vi "标准波形子VI.vi"(4 "采样信息":cluster{"Fs":dbl, "#s":dbl}={"Fs"=1000.0, "#s"=1000.0} {"Fs" format="%.2p"}, 5 "幅值":dbl, 6 "formula":string="sin(w*t)*sin(2*pi(1)*t)" caption="公式", 7 "波形选择":enum16{"正弦波", "三角波", "方波", "锯齿波", "公式波"}(ring), 8 "方波占空比":dbl=50.0 caption="方波占空比(%)" format="%0.2f", 9 "相位":dbl, 11 "频率":dbl) -> (2 "波形图":waveform(dbl)(graph))   [LabVIEW 2017]
uses:
  <vilib>/measure/NI_MABase.lvlib
  <vilib>/measure/NI_MAPro.lvlib
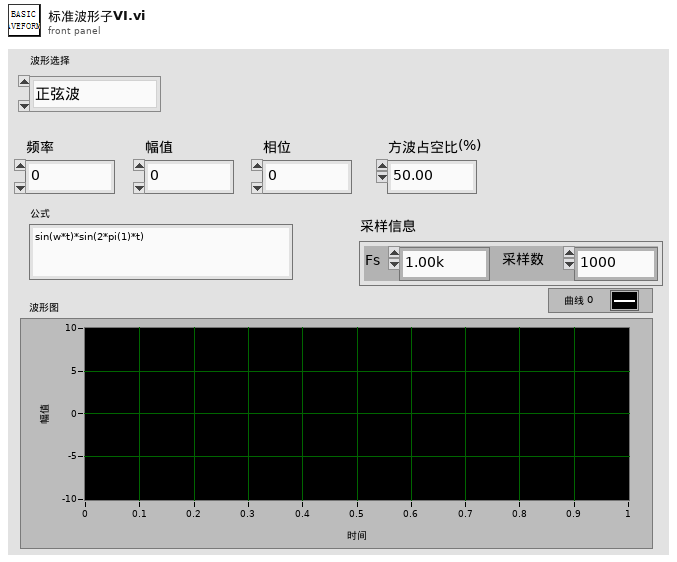
[diagram p1: front panel]
types:
  T1 = enum16{"Sine Wave", "Triangle Wave", "Square Wave", "Sawtooth Wave"}
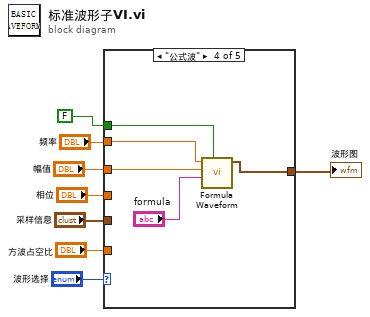
[diagram p0: block diagram]
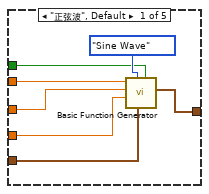
[diagram p2: hidden frame]
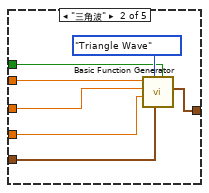
[diagram p3: hidden frame]
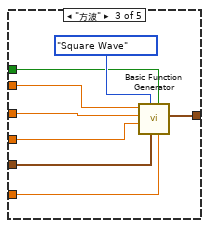
[diagram p4: hidden frame]
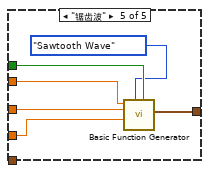
[diagram p5: hidden frame]
diagram:
  n1 = case shown="\"公式波\"" "波形选择" {
    tunnel: [w11 w22 w24 w31 w36] -> w1
    tunnel: "频率" -> [w14 w20 w29 w34 w41]
    tunnel: "幅值" -> [w13 w19 w28 w33 w40]
    tunnel: "相位" -> [w10 w18 w27 _ w39]
    tunnel: "采样信息" -> [w12 w17 w26 _ _]
    tunnel: "方波占空比" -> [_ _ w25 _ _]
    tunnel: FALSE ("reset signal") -> [w9 w16 w23 w35 w38]
    frame "正弦波", Default {
      n2 = call <vilib>:"Basic Function Generator.vi"("reset signal"=w9, "sampling info"=w12, "signal type"=T1."Sine Wave", "phase"=w10, "amplitude"=w13, "frequency"=w14) -> ("signal out"=w11:waveform(dbl))  [unwired: 3 in, 2 out]
    }
    frame "三角波" {
      n3 = call <vilib>:"Basic Function Generator.vi"("reset signal"=w16, "sampling info"=w17, "signal type"=T1."Triangle Wave", "phase"=w18, "amplitude"=w19, "frequency"=w20) -> ("signal out"=w22:waveform(dbl))  [unwired: 3 in, 2 out]
    }
    frame "方波" {
      n4 = call <vilib>:"Basic Function Generator.vi"("square wave duty cycle (%)"=w25, "reset signal"=w23, "sampling info"=w26, "signal type"=T1."Square Wave", "phase"=w27, "amplitude"=w28, "frequency"=w29) -> ("signal out"=w24:waveform(dbl))  [unwired: 2 in, 2 out]
    }
    frame "公式波" {
      n5 = call <vilib>:"Formula Waveform.vi"("reset signal"=w35, "formula"="formula", "amplitude"=w33, "frequency"=w34) -> ("signal out"=w31:waveform(dbl))  [unwired: 6 in, 1 out]
    }
    frame "锯齿波" {
      n6 = call <vilib>:"Basic Function Generator.vi"("reset signal"=w38, "signal type"=T1."Sawtooth Wave", "phase"=w39, "amplitude"=w40, "frequency"=w41) -> ("signal out"=w36:waveform(dbl))  [unwired: 4 in, 2 out]
    }
  }
  "波形图" <- w1
